vi "Test_EmptyBuffer_AvgEquals0.vi"(8 "error in (no error)":errorcluster, 11 "TestCase in":refnum<class "TestTimedAverageBuffer.lvclass">) -> (0 "error out":errorcluster, 3 "TestCase out":refnum<class "TestTimedAverageBuffer.lvclass">)   [LabVIEW 2015, in "TestTimedAverageBuffer.lvclass"]
uses:
  TestTimedAverageBuffer.lvclass
  TimedAverageBuffer.lvclass/TimedAverageBuffer.ctl
  <vilib>/addons/_JKI Toolkits/VI Tester/TestCase.llb/TestCase.lvclass
  TimedAverageBuffer.lvclass
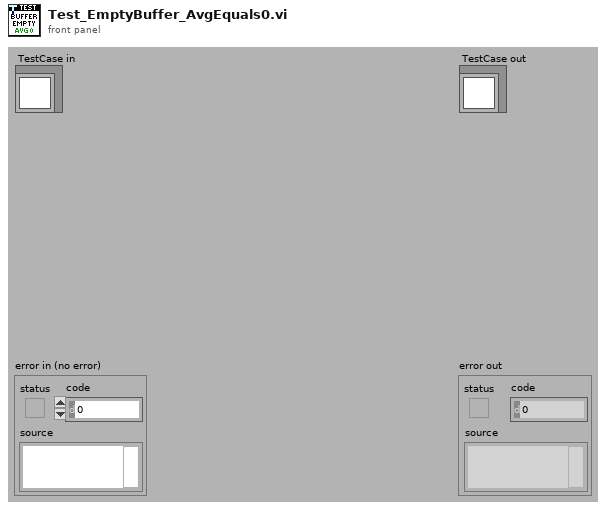
[diagram p1: front panel]
types:
  T1 = typedef "TimedAverageBuffer.lvlib/TimedAverageBuffer.lvclass/TimedAverageBuffer Reference.ctl" = refnum<data-value>
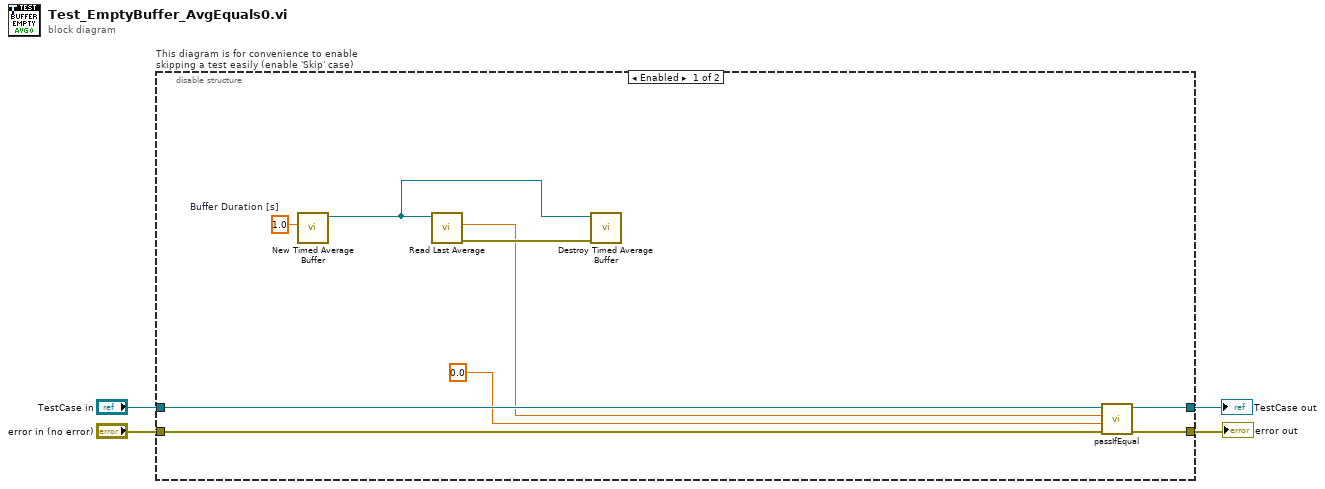
[diagram p0: block diagram]
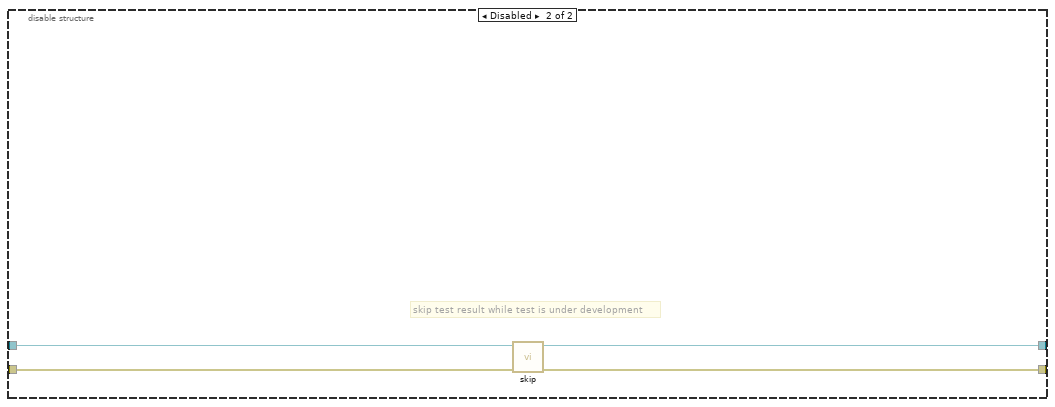
[diagram p2: hidden frame]
diagram:
  n1 = disable-structure "This diagram is for convenience to enable skipping a test easily (enable 'Skip' case)" shown="Enabled" {
    disable-tunnel: "TestCase in" -> [w13 w17]
    disable-tunnel: [w12 w15] -> w1
    disable-tunnel: [w11 w16] -> w3
    disable-tunnel: "error in (no error)" -> [w10 w14]
    frame Enabled {
      w5 = 1.0  # Buffer Duration [s]
      n2 = call "New Timed Average Buffer.vi"("Buffer Duration [s]"=w5) -> ("Timed Average Buffer"=w8:T1)  [unwired: 9 in, 1 out]
      n3 = call "Read Last Average.vi"("Timed Average Buffer"=w8) -> ("error IO"=w7:errorcluster, "Last Average"=w6:dbl)  [unwired: 9 in]
      n4 = call "Destroy Timed Average Buffer.vi"("error in (no error)"=w7, "Timed Average Buffer"=w8) -> ()  [unwired: 9 in, 1 out]
      n5 = call-dynamic "passIfEqual.vi"("error in (no error)"=w10, "y"=0.0, "x"=w6, "TestCase in"=w13) -> ("error out"=w11:errorcluster, "TestCase out"=w12:refnum<class "TestTimedAverageBuffer.lvclass">)  [unwired: 6 in]
    }
    frame Disabled {
      # "skip test result while test is under development"
      n6 = call <vilib>:"skip.vi"("error in (no error)"=w14, "TestCase in"=w17) -> ("error out"=w16:errorcluster, "TestCase out"=w15:refnum<class "TestTimedAverageBuffer.lvclass">)  [unwired: 8 in]
    }
  }
  "error out" <- w3
  "TestCase out" <- w1
